vi "subdev spec pair free.vi"(8 "error in (no error)":errorcluster, 11 "subdev_spec_pair":cluster{"db_name":u64, "sd_name":u64}) -> (0 "error out":errorcluster, 1 "sd_name":string, 2 "db_name":string, 3 "subdev_spec_pair out":cluster{"db_name":u64, "sd_name":u64}, 5 "function return":u32(ring))   [LabVIEW 2023, in "uhd.lvlib"]
doc: "UHD_API uhd_error uhd_subdev_spec_pair_free(uhd_subdev_spec_pair_t* subdev_spec_pair);"
uses:
  <vilib>/Utility/importsl/GetValueByPointer/datatype.ctl
  <vilib>/Utility/importsl/GetValueByPointer/GetValueByPointer.xnode
  <userlib>/uhd/uhd.lvlib
  <userlib>/uhd/uhd.dll
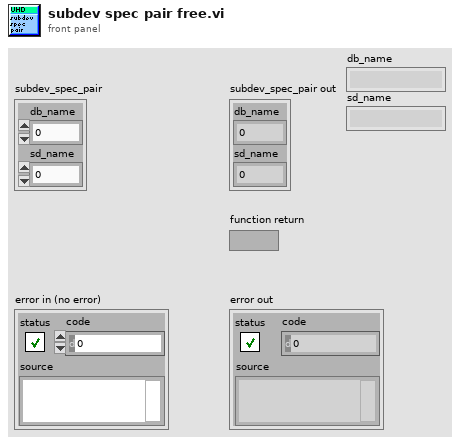
[diagram p1: front panel]
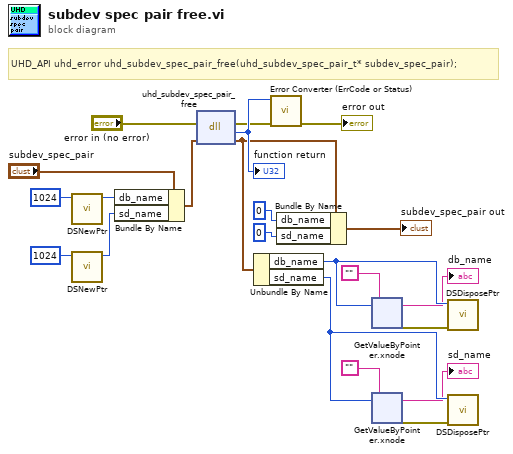
[diagram p0: block diagram]
diagram:
  # "UHD_API uhd_error uhd_subdev_spec_pair_free(uhd_subdev_spec_pair_t* subdev_spec_pair);"
  n1 = call <vilib>:"DSNewPtr.vi"("Size"=u64 1024) -> ("Pointer"=w18:u64)  [unwired: 9 in, 1 out]
  n2 = call <vilib>:"DSNewPtr.vi"("Size"=u64 1024) -> ("Pointer"=w16:u64)  [unwired: 9 in, 1 out]
  n3 = Bundle By Name(cluster="subdev_spec_pair", "db_name"=w18, "sd_name"=w16) -> (w17:cluster{"db_name":u64, "sd_name":u64})
  n4 = dll-call lib="C:/Program Files/National Instruments/LabVIEW 2023/user.lib/uhd/uhd.*" fn="uhd_subdev_spec_pair_free"(error in="error in (no error)", "subdev_spec_pair"=w17) -> (error out=w2:errorcluster, w22:u32, "subdev_spec_pair"=w7:cluster{"db_name":u64, "sd_name":u64})  [unwired: 2 in, 1 out]
  "function return" <- w22
  n5 = Unbundle By Name(w7) -> ("db_name"=w14:u64, "sd_name"=w10:u64)
  n6 = call <userlib>:"Error Converter (ErrCode or Status).vi"("error in (no error)"=w2, "error code"=w22) -> ("error out"=→"error out":errorcluster)  [unwired: 9 in]
  n7 = Bundle By Name(cluster=w7, "db_name"=u64 0, "sd_name"=u64 0) -> (→"subdev_spec_pair out":cluster{"db_name":u64, "sd_name":u64})
  n8 = xnode "GetValueByPointer.xnode"("Pointer"=w14, "InputType"="") -> ("Output"=→"db_name":string, "ErrorOut"=w15:errorcluster)  [unwired: 2 in]
  n9 = xnode "GetValueByPointer.xnode"("Pointer"=w10, "InputType"="") -> ("Output"=→"sd_name":string, "ErrorOut"=w11:errorcluster)  [unwired: 2 in]
  n10 = call <vilib>:"DSDisposePtr.vi"("error in (no error)"=w15, "Pointer"=w14) -> ()  [unwired: 9 in, 1 out]
  n11 = call <vilib>:"DSDisposePtr.vi"("error in (no error)"=w11, "Pointer"=w10) -> ()  [unwired: 9 in, 1 out]
